vi "GetEvents.vi"(8 "error in (no error)":errorcluster, 11 "CameraI2CUSB in":refnum<class "CameraSim.lvclass">) -> (0 "error out":errorcluster, 2 "Events":T1, 3 "CameraI2CUSB out":refnum<class "CameraSim.lvclass">)   [LabVIEW 2020, in "CameraSim.lvlib" / "CameraSim.lvclass"]
doc: "Return events generates from camera"
uses:
  CameraSim.lvclass
  CameraSim.lvclass/CameraSim.ctl
  ICamera/ICamera/TypeDef/Events.ctl
  ICamera/ICamera/ICamera.lvclass
  ICamera/ICamera/TypeDef/StreamDataEvent.ctl
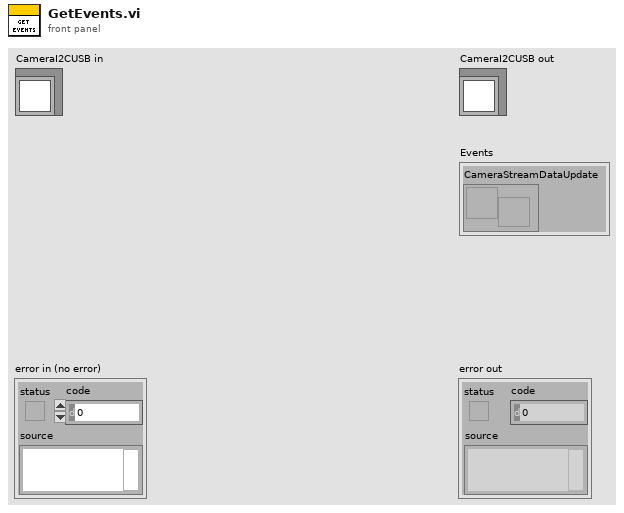
[diagram p1: front panel]
types:
  T1 = typedef "ICamera.lvlib/ICamera.lvclass/Events.ctl" = cluster{"CameraStreamDataUpdate":T2}
  T2 = typedef "ICamera.lvlib/ICamera.lvclass/StreamDataEvent.ctl" = refnum<user-event>
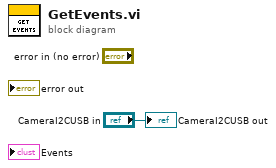
[diagram p0: block diagram]
diagram:
  "CameraI2CUSB out" <- "CameraI2CUSB in"
